vi "Abort Sequence Load-Single.vi"(8 "error in":errorcluster, 11 "Abort Sequence - Single":T1) -> (0 "error out":errorcluster)   [LabVIEW 2021]
doc: "Abort the sequence and if error resets the device."
uses:
  controls/Abort Sequence-Single.ctl
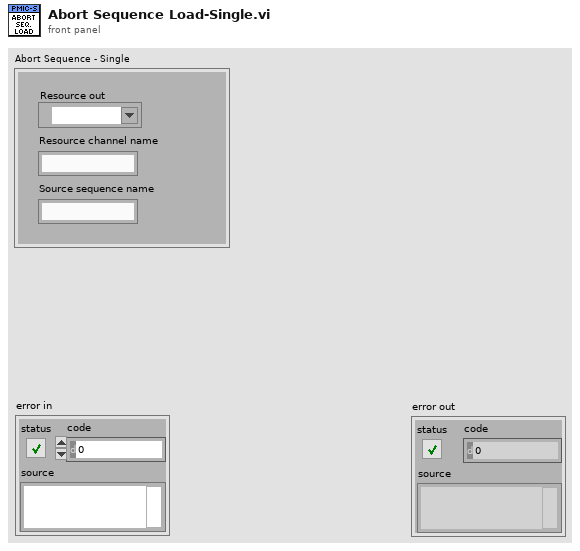
[diagram p1: front panel]
types:
  T1 = typedef "Abort Sequence-Single.ctl" = cluster{"Resource out":refnum<k15>, "Resource channel name":string, "Source sequence name":string}
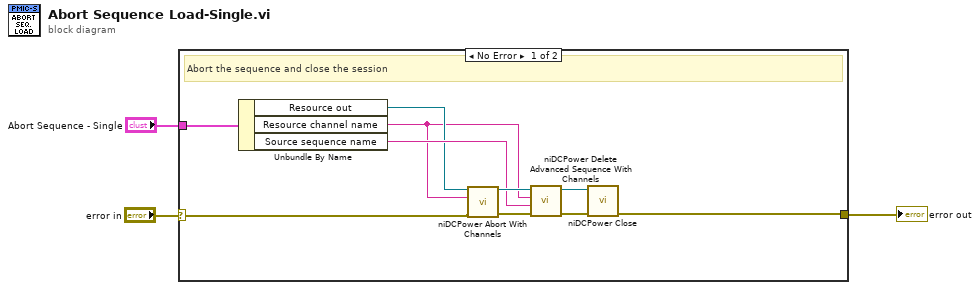
[diagram p0: block diagram]
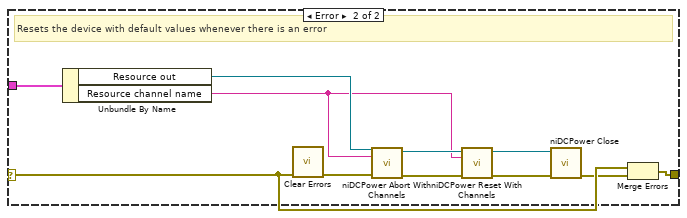
[diagram p2: hidden frame]
diagram:
  n1 = case shown="No Error" "error in" {
    selector: "error in" -> [w4 w16]
    tunnel: "Abort Sequence - Single" -> [w13 w24]
    tunnel: [w5 w14] -> w1
    frame No Error {
      # "Abort the sequence and close the session"
      n2 = Unbundle By Name(w13) -> ("Resource out"=w7:refnum<k15>, "Resource channel name"=w6:string, "Source sequence name"=w8:string)
      n3 = call <instrlib>:"niDCPower Abort With Channels.vi"("error in (no error)"=w4, "channel name"=w6, "instrument handle"=w7) -> ("error out"=w12:errorcluster, "instrument handle out"=w11:refnum<k15>)  [unwired: 7 in]
      n4 = call <instrlib>:"niDCPower Delete Advanced Sequence With Channels.vi"("error in (no error)"=w12, "sequence name"=w8, "channel name"=w6, "instrument handle"=w11) -> ("error out"=w10:errorcluster, "instrument handle out"=w9:refnum<k15>)  [unwired: 6 in]
      n5 = call <instrlib>:"niDCPower Close.vi"("error in (no error)"=w10, "instrument handle"=w9) -> ("error out"=w5:errorcluster)  [unwired: 9 in]
    }
    frame Error {
      # "Resets the device with default values whenever there is an error"
      n6 = Unbundle By Name(w24) -> ("Resource out"=w19:refnum<k15>, "Resource channel name"=w18:string)
      n7 = call <vilib>:"Clear Errors.vi"("error in (no error)"=w16) -> ("error out"=w17:errorcluster)  [unwired: 5 in, 1 out]
      n8 = call <instrlib>:"niDCPower Abort With Channels.vi"("error in (no error)"=w17, "channel name"=w18, "instrument handle"=w19) -> ("error out"=w23:errorcluster, "instrument handle out"=w22:refnum<k15>)  [unwired: 7 in]
      n9 = call <instrlib>:"niDCPower Reset With Channels.vi"("error in (no error)"=w23, "channel name"=w18, "instrument handle"=w22) -> ("error out"=w21:errorcluster, "instrument handle out"=w20:refnum<k15>)  [unwired: 7 in]
      n10 = call <instrlib>:"niDCPower Close.vi"("error in (no error)"=w21, "instrument handle"=w20) -> ("error out"=w15:errorcluster)  [unwired: 9 in]
      n11 = Merge Errors(w16, w15) -> (w14:errorcluster)
    }
  }
  "error out" <- w1
